vi "Write path.vi"(8 "error in (no error)":errorcluster, 10 "path":string, 11 "WebsocketsConnection in":refnum<class "WebsocketsConnection.lvclass">) -> (0 "error out":errorcluster, 3 "WebsocketsConnection out":refnum<class "WebsocketsConnection.lvclass">)   [LabVIEW 2013, in "MQTT_Websockets.lvlib" / "WebsocketsConnection.lvclass"]
uses:
  WebsocketsConnection.lvclass
  WebsocketsConnection.lvclass/WebsocketsConnection.ctl
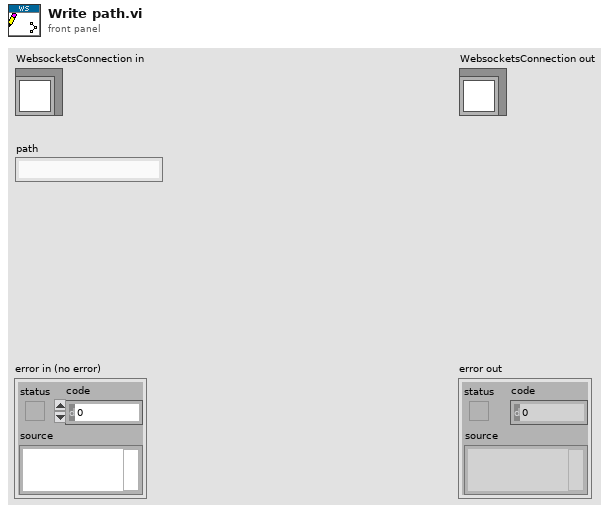
[diagram p1: front panel]
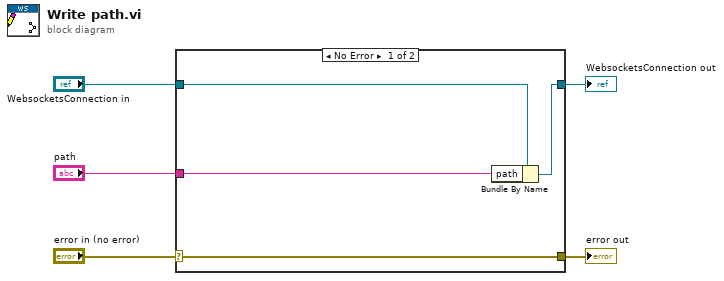
[diagram p0: block diagram]
diagram:
  n1 = case shown="No Error" "error in (no error)" {
    selector: "error in (no error)" -> [w9 w10]
    tunnel: [w9 w10] -> w4
    tunnel: [w7 w11] -> w2
    tunnel: "WebsocketsConnection in" -> [w8 w11]
    tunnel: "path" -> [w6 _]
    frame No Error {
      n2 = Bundle By Name(cluster=w8, "path"=w6) -> (w7:refnum<class "WebsocketsConnection.lvclass">)
    }
    frame Error {
    }
  }
  "error out" <- w4
  "WebsocketsConnection out" <- w2
